vi "filterReferee.vi"(6 "Command":string, 8 "error in (no error)":errorcluster, 10 "RefBox UDP RX":T2, 11 "Vision in":refnum<class "Vision.lvclass">) -> (0 "error out":errorcluster, 1 "SSL Referee Game Status":T1 {"Time" format="%<%.3X %x>T"; "Blue Timeout Remaining" format="%<%M:%S>t"; "Yellow Timeout Remaining" format="%<%M:%S>t"; "Time Left" format="%<%M:%S>t"}, 2 "GUI Game Status":T1 {"Time" format="%<%.3X %x>T"; "Blue Timeout Remaining" format="%<%M:%S>t"; "Yellow Timeout Remaining" format="%<%M:%S>t"; "Time Left" format="%<%M:%S>t"}, 3 "Vision out":refnum<class "Vision.lvclass">, 5 "RX":bool)   [LabVIEW 2018, in "Vision.lvclass"]
uses:
  Vision.lvclass
  Controls/vision_control.ctl
  Old vision/Decode SSL and Refree Wrapper Package Folder/SSL Referee Game Status.ctl
panel:
  # "Score"
  # "Red Cards"
  # "Yellow Cards"
  # "Timeouts Left"
  # "Timeout Remaining"
  # "Goalie ID"
  # "Score"
  # "Red Cards"
  # "Yellow Cards"
  # "Timeouts Left"
  # "Timeout Remaining"
  # "Goalie ID"
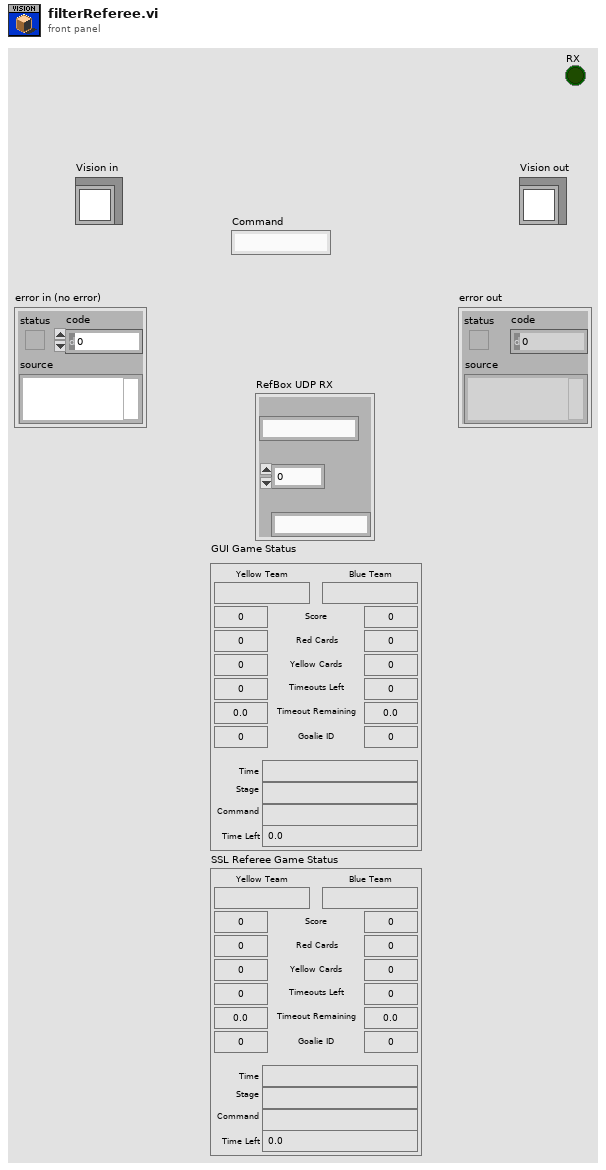
[diagram p1: front panel]
types:
  T1 = typedef "SSL Referee Game Status.ctl" = cluster{"Stage":string, "Command":string, "Time Left":dbl, "Yellow Team":string, "Blue Team":string, "Yellow Score":u32, "Blue Score":u32, "Yellow Red Cards":u32, "Blue Red Cards":u32, "Yellow Yellow Cards":u32, "Blue Yellow Cards":u32, "Yellow Timeouts Left":u32, "Blue Timeouts Left":u32, "Yellow Timeout Remaining":dbl, "Blue Timeout Remaining":dbl, "Yellow Goalie Id":u32, "Blue Goalie Id":u32, "Time":timestamp}
  T2 = typedef "vision_control.ctl" = cluster{"Local IP:":string, "Port":i32, "Server IP:":string}
  T3 = typedef "SSL Referee.ctl" = cluster{"packet_\ntimestamp":u64, "stage":u64, "stage_time_left":i32, "command ":u64, "command_\ncounter ":u32, "command_\ntimestamp":u64, "yellow team info":T4, "blue team info":T4, "Point":cluster{"x":sgl, "y":sgl}}
  T4 = typedef "SSL Referee Team Info.ctl" = cluster{"name":string, "score":u32, "red_cards":u32, "yellow_cards_time":u32[], "yellow_cards":u32, "timeout":u32, "timeout_times":u32, "goalie":u32}
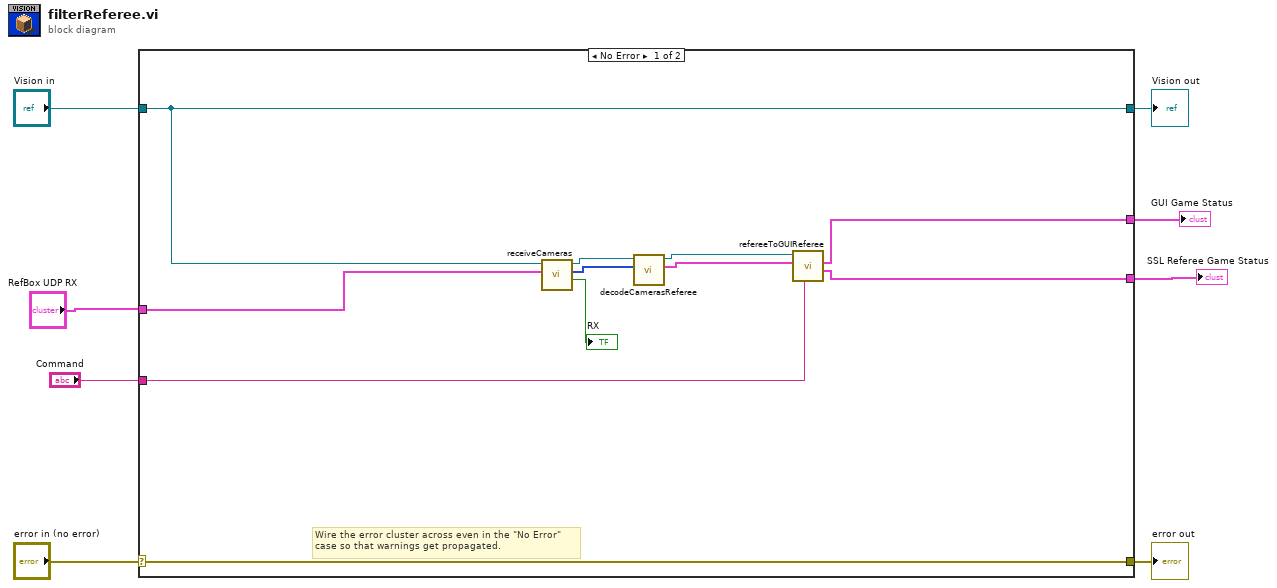
[diagram p0: block diagram]
diagram:
  n1 = case shown="No Error" "error in (no error)" {
    selector: "error in (no error)" -> [w19 w21]
    tunnel: [w19 w21] -> w7
    tunnel: [w13 w20] -> w5
    tunnel: "Vision in" -> [w13 w20]
    tunnel: "RefBox UDP RX" -> [w14 _]
    tunnel: [w12 _] -> w3
    tunnel: [w11 _] -> w2
    tunnel: "Command" -> [w10 _]
    frame No Error {
      # "Wire the error cluster across even in the \"No Error\"\ncase so that warnings get propagated."
      n2 = call "receiveCameras.vi"("Cluster"=w14, "Vision in"=w13) -> ("RX"=→"RX":bool, "data camera out"=w17:u8[], "Vision out"=w15:refnum<class "Vision.lvclass">)  [unwired: 5 in, 1 out]
      n3 = call "decodeCamerasReferee.vi"("element"=w17, "Vision in"=w15) -> ("SSL Game Status"=w18:T3, "Vision out"=w16:refnum<class "Vision.lvclass">)  [unwired: 7 in, 1 out]
      n4 = call "refereeToGUIReferee.vi"("Command"=w10, "SSL Game Status"=w18, "Vision in"=w16) -> ("SSL Referee Game Status"=w11:T1, "GUI Game Status"=w12:T1)  [unwired: 5 in, 2 out]
    }
    frame Error {
    }
  }
  "error out" <- w7
  "Vision out" <- w5
  "GUI Game Status" <- w3
  "SSL Referee Game Status" <- w2
